vi "HomeCMD.vi"(8 "error in (no error)":errorcluster, 11 "ThorlabsLabJack in":refnum<class "ThorlabsLabJack.lvclass">) -> (0 "error out":errorcluster, 3 "ThorlabsLabJack out":refnum<class "ThorlabsLabJack.lvclass">)   [LabVIEW 2018, in "ThorlabsLabJack.lvlib" / "ThorlabsLabJack.lvclass"]
uses:
  ThorlabsLabJack.lvclass
  ThorlabsLabJack.lvclass/ThorlabsLabJack.ctl
  C:/AME Test Engineering/LabVIEW/PPLs/Axis/Thorlabs/Thorlabs.MotionControl.IntegratedStepperMotorsCLI.dll
  PPLs/Axis/Thorlabs/Thorlabs.MotionControl.IntegratedStepperMotorsCLI.dll
  a5d5979f-18be-4e82-98d2-e3e3f93858e8.vi
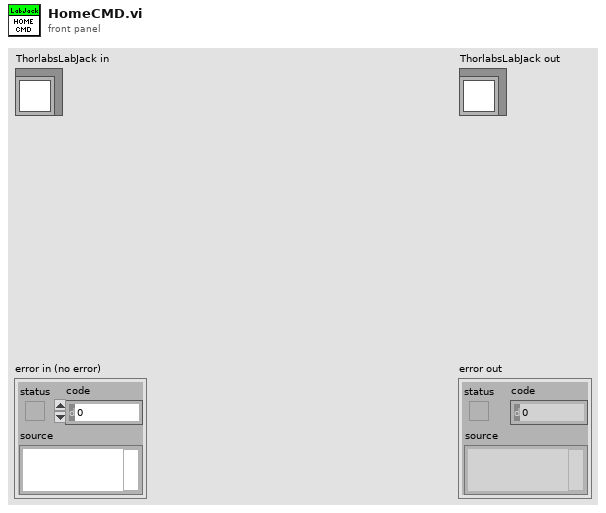
[diagram p1: front panel]
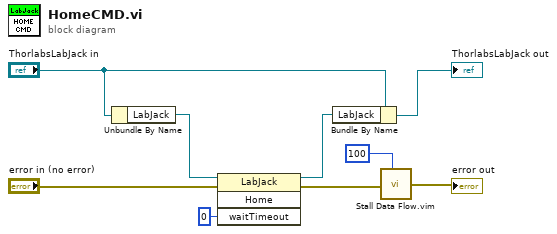
[diagram p0: block diagram]
diagram:
  n1 = Unbundle By Name("ThorlabsLabJack in") -> ("LabJack"=w8:refnum<k24>)
  n2 = invoke class="LabJack" method="Home"(reference=w8, error in="error in (no error)", "waitTimeout"=0) -> (reference out=w7:refnum<k24>, error out=w2:errorcluster)  [unwired: 1 in, 2 out]
  n3 = Bundle By Name(cluster="ThorlabsLabJack in", "LabJack"=w7) -> (→"ThorlabsLabJack out":refnum<class "ThorlabsLabJack.lvclass">)
  n4 = call "Stall Data Flow.vim"("value in"=w2, "milliseconds to wait"=u32 100) -> ("value out"=→"error out":errorcluster)  [unwired: 1 out]
